vi "runLoadSummaryByManual.vi"() -> ()   [LabVIEW 2012]
panel:
  out "error out":errorcluster
  out "Message":string
  out "目錄":path
  out "Files":string
  in  "OK Button":bool
  in  "stop":bool
  in  "1.請先選檔案目錄":path
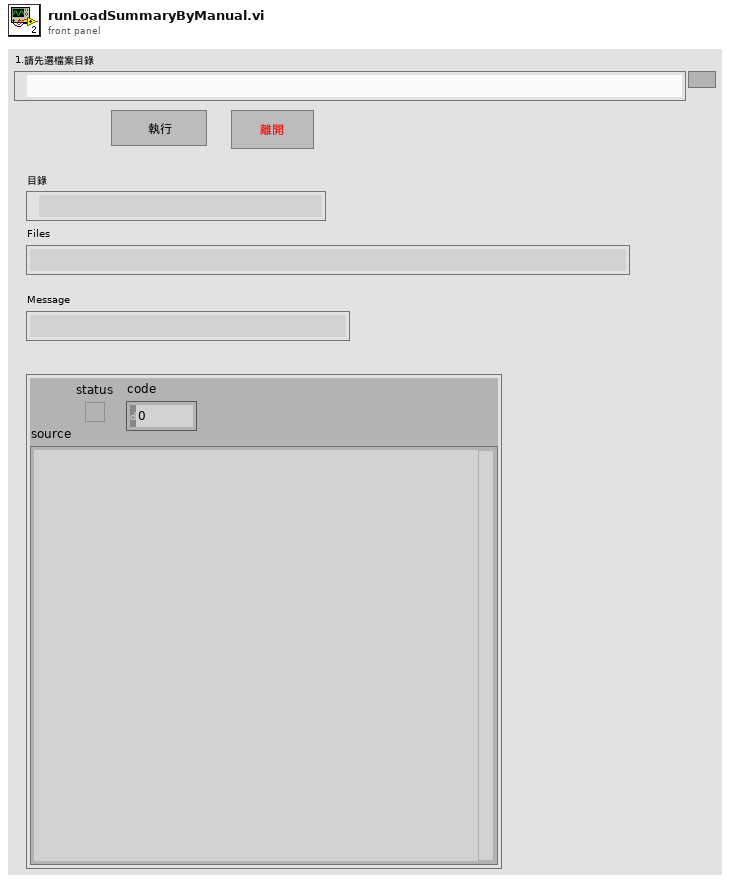
[diagram p1: front panel]
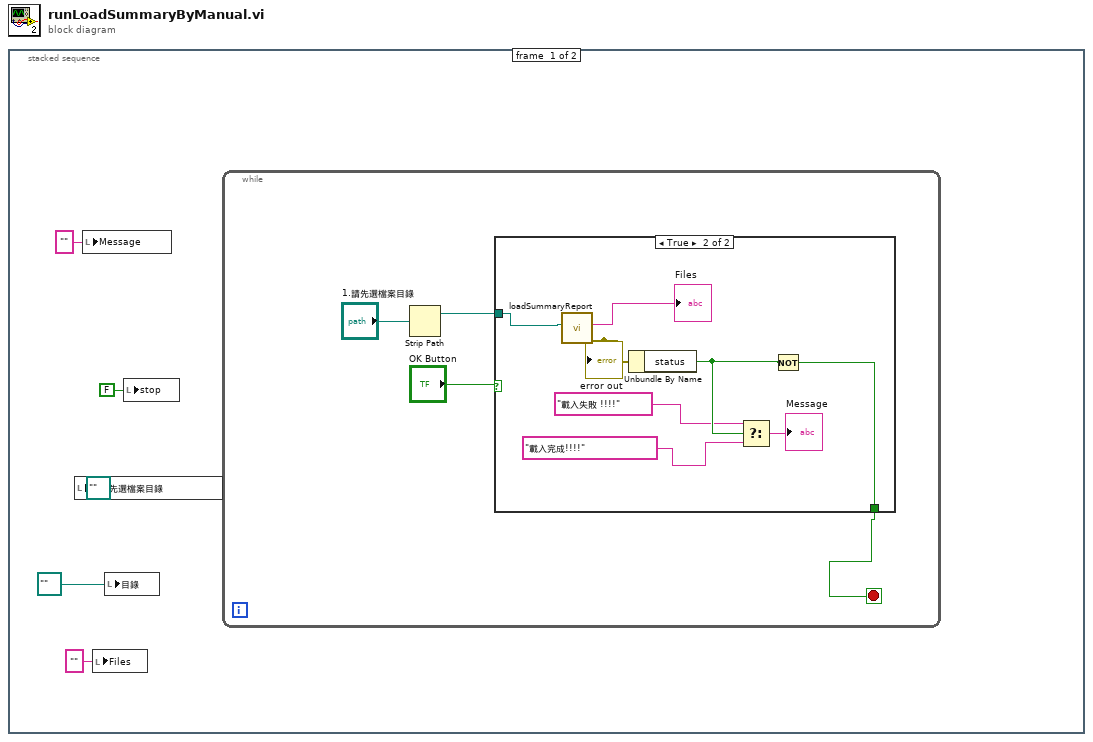
[diagram p0: block diagram]
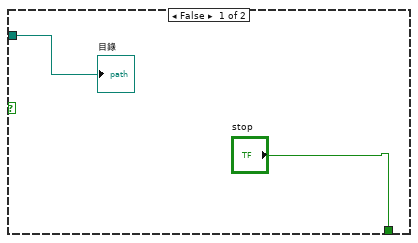
[diagram p2: hidden frame]
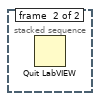
[diagram p3: hidden frame]
diagram:
  n1 = stacked-sequence {
    frame #0 {
      n2 = local write "1.請先選檔案目錄"(path "" ("Path")) -> ()
      n3 = local write "Message"("" ("Message")) -> ()
      n4 = local write "Files"("" ("Files")) -> ()
      n5 = local write "目錄"(path "" ("stripped path")) -> ()
      n6 = local write "stop"(FALSE ("stop")) -> ()
      n7 = while {
        stop <- w6 stop-if-true
        n8 = Strip Path(path="1.請先選檔案目錄") -> (stripped path=w7:path)  [unwired: 1 out]
        n9 = case shown="True" "OK Button" {
          tunnel: w7 -> [w10 w19]
          tunnel: ["stop" w16] -> w6
          frame False {
            "目錄" <- w10
          }
          frame True {
            n10 = call "loadSummaryReport.vi"("path"=w19) -> ("error out"=w17:errorcluster, "Files"=→"Files":string)  [unwired: 9 in]
            "error out" <- w17
            n11 = Unbundle By Name(w17) -> ("status"=w15:bool)
            n12 = Select(t="載入失敗 !!!!", s=w15, f="載入完成!!!!") -> (s? t:f=→"Message":string)
            n13 = Not(x=w15) -> (.not. x?=w16:bool)
          }
        }
      }
    }
    frame #1 {
      n14 = Quit LabVIEW() -> ()  [unwired: 1 in]
    }
  }
